vi "Read Bus Load Settings.vi"(8 "error in (no error)":errorcluster, 11 "Port Ref in":T2 format="%.0x") -> (0 "error out":errorcluster, 2 "Bus Load Settings":T1, 3 "Port Ref out":T2 format="%.0x")   [LabVIEW 2018, in "NI-XNET Monitor System Explorer.lvlib"]
uses:
  NI-XNET Monitor System Explorer.lvlib
  <vilib>/NI Veristand/Custom Device API/Custom Device Item Ref.ctl
  Shared/BusLoad.Settings.ctl
  Shared/Constants.vi
  <vilib>/NI Veristand/Custom Device API/Get Item Property (Boolean).vi
  <vilib>/NI Veristand/Custom Device API/Get Item Property (U32).vi
  <vilib>/NI Veristand/Custom Device API/Custom Device API.lvlib
  Shared/NI-XNET Monitor Shared.lvlib
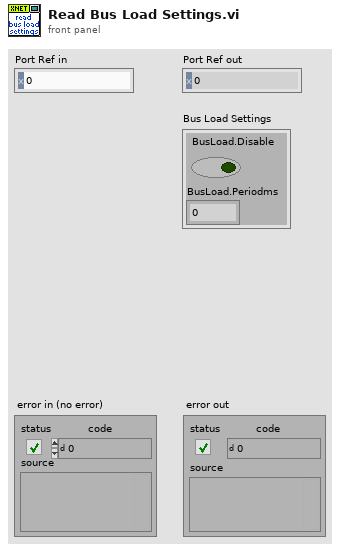
[diagram p1: front panel]
types:
  T1 = typedef "NI-XNET Monitor Shared.lvlib/BusLoad.Settings.ctl" = cluster{"BusLoad.Disable":bool, "BusLoad.Periodms":u32}
  T2 = typedef "Custom Device API.lvlib/Custom Device Item Ref.ctl" = u64
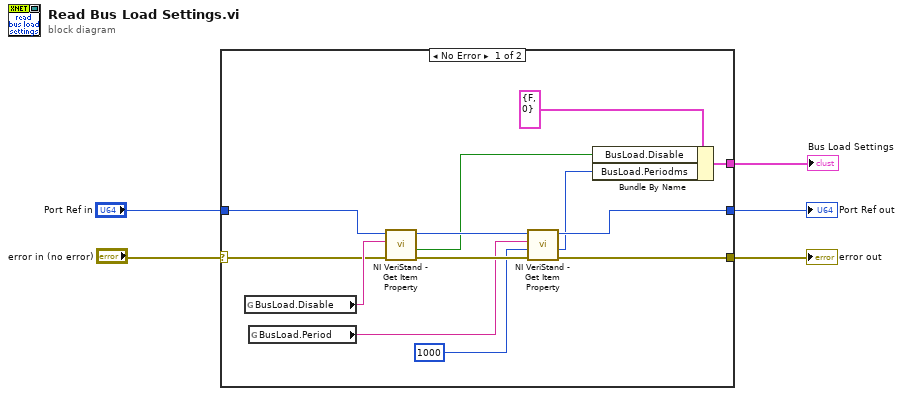
[diagram p0: block diagram]
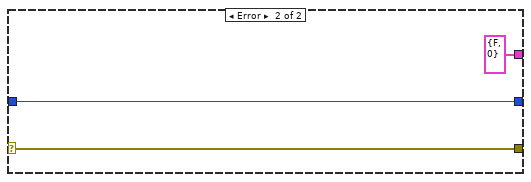
[diagram p2: hidden frame]
diagram:
  n1 = case shown="No Error" "error in (no error)" {
    selector: "error in (no error)" -> [w12 w20]
    tunnel: [w13 w20] -> w5
    tunnel: "Port Ref in" -> [w11 w21]
    tunnel: [w10 w21] -> w2
    tunnel: [w6 T1 {"BusLoad.Disable"=FALSE, "BusLoad.Periodms"=0} ("Bus Load Settings")] -> w1
    frame No Error {
      n2 = global read "Constants.vi" "BusLoad.Disable"() -> (w18:string)
      n3 = global read "Constants.vi" "BusLoad.Period"() -> (w15:string)
      n4 = call-poly <vilib>:"NI VeriStand - Get Item Property.vi"("error in (no error)"=w12, "Property Name"=w18, "Item Ref in"=w11) -> ("error out"=w16:errorcluster, "Value"=w8:bool, "Item Ref out"=w17:T2)  [unwired: 5 in, 1 out]
      n5 = call-poly <vilib>:"NI VeriStand - Get Item Property.vi"("error in (no error)"=w16, "Default Value"=u32 1000, "Property Name"=w15, "Item Ref in"=w17) -> ("error out"=w13:errorcluster, "Value"=w7:u32, "Item Ref out"=w10:T2)  [unwired: 4 in, 1 out]
      n6 = Bundle By Name(cluster=T1 {"BusLoad.Disable"=FALSE, "BusLoad.Periodms"=0} ("Bus Load Settings"), "BusLoad.Disable"=w8, "BusLoad.Periodms"=w7) -> (w6:T1)
    }
    frame Error {
    }
  }
  "error out" <- w5
  "Port Ref out" <- w2
  "Bus Load Settings" <- w1
